vi "beginTableWithStrikerPlay.vi"(10 "Game":refnum<class "Game.lvclass">, 11 "TableWithStrikerPlay in":refnum<class "TableWithStrikerPlay.lvclass">) -> (2 "BeginTableWithStriker?":bool, 3 "TableWithStrikerPlay out":refnum<class "TableWithStrikerPlay.lvclass">)   [LabVIEW 2023, in "TableWithStrikerPlay.lvclass"]
uses:
  TableWithStrikerPlay.lvclass
  Game_class/Game.lvclass
  Referee_class/command_interpreted.ctl
  Team_class/OffensivePlay.ctl
  Game_class/Game.lvclass/Game.ctl
  Team_class/Team.lvclass/Team.ctl
  Referee_class/Referee.lvclass/Referee.ctl
  Game_class/Read Referee.vi
  Game_class/Read Utilities.lvclass.vi
  Referee_class/Read command_interpreted.vi
  Game_class/Read OffensiveTeam.vi
  Team_class/Read RobotRef.vi
  Team_class/Read OffensivePlay.vi
  Ally_class/Ally.lvclass
  C:/Users/ebert/Desktop/roboime/SSL_AI/Team_class/Team.lvclass
  Robot_class/Robot.lvclass
  Referee_class/Referee.lvclass
  Utilities_class/Utilities.lvclass
panel:
  out "error out":errorcluster
  in  "error in (no error)":errorcluster
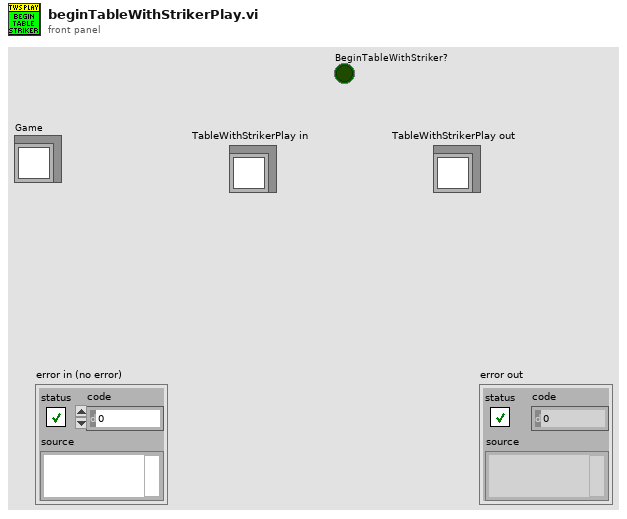
[diagram p1: front panel]
types:
  T1 = typedef "command_interpreted.ctl" = enum16{"Goal Ally", "Goal Enemy", "Ball Placement Enemy", "Ball Placement Ally", "Normal Half Time", "Extra Time  Break", "Extra Half Time", "None", "Post Game", "PKA Normal Start", "Prepare Kickoff Ally", "PKE Normal Start", "Prepare Kickoff Enemy", "Force Start", "Halt", "Timeout", "Prepare Penalty Ally", "Prepare Penalty Enemy", "PPA NormalStart", "PPE Normal Start", "Indirect Free Ally", "Direct Free Enemy", "Direct Free Ally", "Indirect Free Enemy", "Stop"}
  T2 = typedef "OffensivePlay.ctl" = enum16{"5RobotsPassGamePlay", "5PreparePassGame", "5RobotsKeeperGame", "KeeperPassToStriker", "5RobotsNormalGamePlay", "PrepareKeeperPass", "ACBPass", "ABCPass", "PrepareTriplePass", "TableWithStriker", "TableWith2ndStrikerPlay", "PrepareDoublePass", "PrepareRollToPass", "SimplePass", "PreparePass", "PassToStriker", "BallOutOfField", "PassTo2ndStriker", "StopOffensive", "Prepare Penalty Enemy", "EnemyPossessionAtEnemyField", "EnemyPossesionAtOurField", "TestPlay", "PreparePenaltyAlly", "KickPenaltyAlly", "PrepareKickoffAlly", "PrepareKickoffEnemy", "IndirectEnemy", "DirectEnemy", "PreparePassInGame1", "NormalGame", "DirectKick", "Pass", "Halt", "Timeout", "PassPlay", "PenaltyEnemy"}
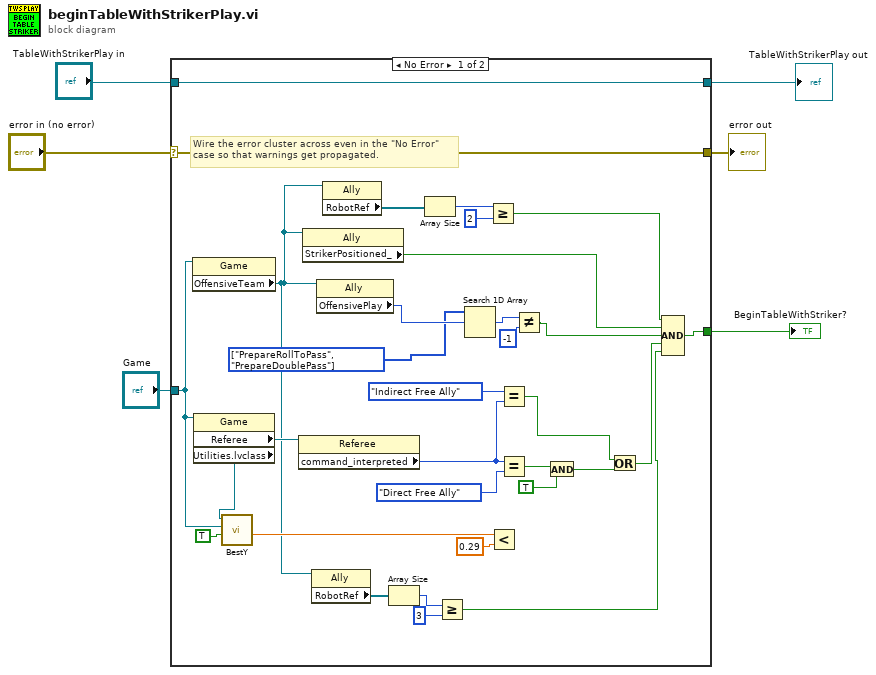
[diagram p0: block diagram]
diagram:
  n1 = case shown="No Error" "error in (no error)" {
    selector: "error in (no error)" -> [w37 w40]
    tunnel: [w37 w40] -> w5
    tunnel: [w38 w39] -> w1
    tunnel: "TableWithStrikerPlay in" -> [w38 w39]
    tunnel: "Game" -> [w29 _]
    tunnel: [w28 _] -> w3
    frame No Error {
      w9 = T2[] [enum."PrepareRollToPass", enum."PrepareDoublePass"] items=["5RobotsPassGamePlay", "5PreparePassGame", "5RobotsKeeperGame", "KeeperPassToStriker", "5RobotsNormalGamePlay", "PrepareKeeperPass", "ACBPass", "ABCPass", "PrepareTriplePass", "TableWithStriker", "TableWith2ndStrikerPlay", "PrepareDoublePass", "PrepareRollToPass", "SimplePass", "PreparePass", "PassToStriker", "BallOutOfField", "PassTo2ndStriker", "StopOffensive", "Prepare Penalty Enemy", "EnemyPossessionAtEnemyField", "EnemyPossesionAtOurField", "TestPlay", "PreparePenaltyAlly", "KickPenaltyAlly", "PrepareKickoffAlly", "PrepareKickoffEnemy", "IndirectEnemy", "DirectEnemy", "PreparePassInGame1", "NormalGame", "DirectKick", "Pass", "Halt", "Timeout", "PassPlay", "PenaltyEnemy"] ("Array")
      # "Wire the error cluster across even in the \"No Error\"\ncase so that warnings get propagated."
      n2 = property class="Game"(reference=w29) -> ("OffensiveTeam"=w15:refnum<class "Ally.lvclass">)  [unwired: 1 in, 2 out]
      n3 = property class="Game"(reference=w29) -> ("Referee"=w36:refnum<class "Referee.lvclass">, "Utilities.lvclass"=w19:refnum<class "Utilities.lvclass">)  [unwired: 1 in, 2 out]
      n4 = call "BestY.vi"("Utilities in"=w19, "Game"=w29, "inimigos"=TRUE) -> ("Gap kick"=w30:dbl)  [unwired: 2 in, 4 out]
      n5 = property class="Referee"(reference=w36) -> ("command_interpreted"=w34:T1)  [unwired: 1 in, 2 out]
      n6 = property class="Ally"(reference=w15) -> ("StrikerPositioned_"=w27:bool)  [unwired: 1 in, 2 out]
      n7 = property class="Ally"(reference=w15) -> ("RobotRef"=w18:refnum<class "Robot.lvclass">[])  [unwired: 1 in, 2 out]
      n8 = property class="Ally"(reference=w15) -> ("OffensivePlay"=w10:T2)  [unwired: 1 in, 2 out]
      n9 = property class="Ally"(reference=w15) -> ("RobotRef"=w24:refnum<class "Robot.lvclass">[])  [unwired: 1 in, 2 out]
      n10 = Array Size(array=w18) -> (size(s)=w17:i32)
      n11 = Array Size(array=w24) -> (size(s)=w23:i32)
      n12 = Greater Or Equal?(x=w17, y=3) -> (x >= y?=w14:bool)
      n13 = Search 1D Array(1D array=w9, element=w10) -> (index of element=w13:i32)  [unwired: 1 in]
      n14 = Greater Or Equal?(x=w23, y=2) -> (x >= y?=w21:bool)
      n15 = Less?(x=w30, y=0.29 ("Gap kick")) -> ()  [unwired: 1 out]
      n16 = Equal?(x=command_interpreted."Indirect Free Ally" ("command_interpreted"), y=w34) -> (x = y?=w25:bool)
      n17 = Equal?(x=w34, y=command_interpreted."Direct Free Ally" ("command_interpreted")) -> (x = y?=w26:bool)
      n18 = Not Equal?(x=w13, y=-1) -> (x != y?=w11:bool)
      n19 = And(x=w26, y=TRUE) -> (x .and. y?=w8:bool)
      n20 = Or(x=w25, y=w8) -> (x .or. y?=w20:bool)
      n21 = Compound Arithmetic op=AND(w21, w27, w11, w20, w14) -> (w28:bool)
    }
    frame Error {
    }
  }
  "error out" <- w5
  "BeginTableWithStriker?" <- w3
  "TableWithStrikerPlay out" <- w1
